vi "Module Name--constant.vi"() -> (3 "Module Name":string)   [LabVIEW 2020, in "S7.lvlib"]
doc: "Return the name of the module that owns this VI. \n_____\nBased on Delacor QMH Project Template 4.1.0.59."
uses:
  S7.lvlib
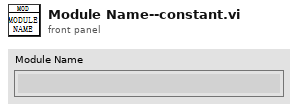
[diagram p1: front panel]
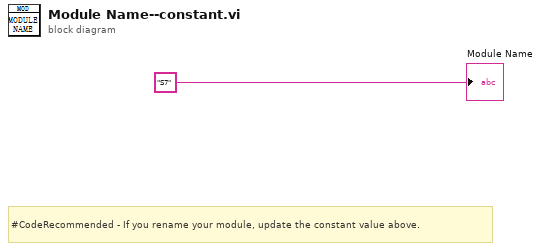
[diagram p0: block diagram]
diagram:
  # "#CodeRecommended - If you rename your module, update the constant value above."
  "Module Name" <- "S7"
